vi "Rd Wr HK Settings.vi"(8 "error in (no error)":errorcluster, 9 "File Path":path, 10 "Write? (F:Read)":bool, 11 "channels":T1[](array[typedef])) -> (0 "error out":errorcluster, 3 "channels":T1[](array[typedef]))   [LabVIEW 2024, in "HK Table.lvclass"]
uses:
  HK Table.lvclass
  HK Channel Settings.ctl
  HK Item/HK Channel Units and Setup.ctl
  HK Item/HK Channel enum Data Type.ctl
  HK Item/HK Channel Settings Scaling.ctl
  HK Item/HK Channel enum Scaling Type.ctl
  HK Item/HK Channel Settings Physical.ctl
  HK Item/HK Channel Settings Limits.ctl
  HK Alarms/HK Channel Settings Alarms.ctl
  HK Alarms/HK Alarm enum Action.ctl
  5f5682ec-8197-494c-a0e5-daa0ddab1ed8.vi
  8967ee68-6fb9-484b-9a6b-7567600e0f71.vi
  <vilib>/JDP Science/JSONtext/JSON text to Variant.vi
  <vilib>/JDP Science/JSONtext/Variant to JSON Text.vi
  <vilib>/JDP Science/JSONtext/LVClass Serializer/JSONtext LVClass Serializer.lvclass
  HK Item/HK Item.lvclass
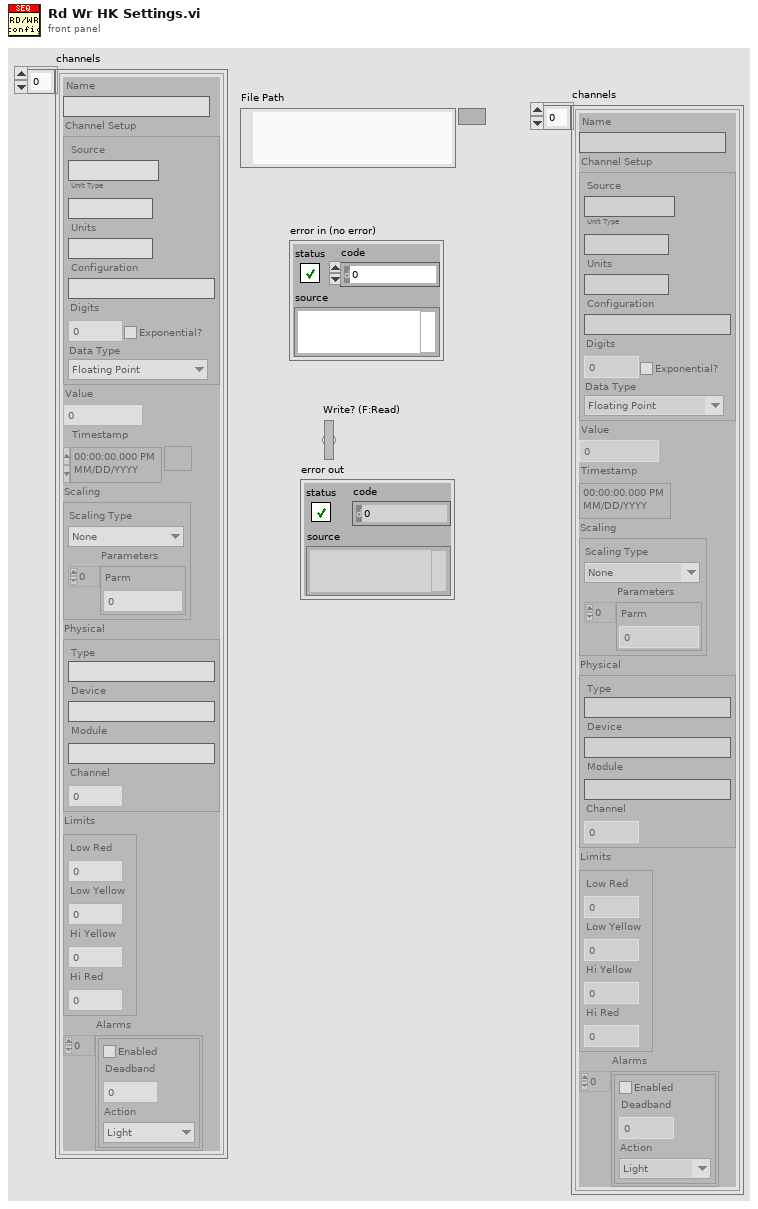
[diagram p1: front panel]
types:
  T1 = typedef "HK Table.lvclass/HK Channel Settings.ctl" = cluster{"Name":string, "Channel Setup":T2, "Value":dbl, "Timestamp":timestamp, "Scaling":T4, "Physical":T6, "Limits":T7, "Alarms":T8[]}
  T2 = typedef "HK Item.lvclass/HK Channel Units and Setup.ctl" = cluster{"Unit Type":string, "Units":string, "Configuration":string, "Digits":i32, "Data Type":T3, "Exponential?":bool, "Source":string}
  T3 = typedef "HK Item.lvclass/HK Channel enum Data Type.ctl" = enum16{"Floating Point", "Integer", "Enum", "String", "Waveform", "File"}
  T4 = typedef "HK Item.lvclass/HK Channel Settings Scaling.ctl" = cluster{"Scaling Type":T5, "Parameters":dbl[]}
  T5 = typedef "HK Item.lvclass/HK Channel enum Scaling Type.ctl" = enum16{"None", "Polynomial"}
  T6 = typedef "HK Item.lvclass/HK Channel Settings Physical.ctl" = cluster{"Type":string, "Device":string, "Module":string, "Channel":i32}
  T7 = typedef "HK Item.lvclass/HK Channel Settings Limits.ctl" = cluster{"Low Red":dbl, "Low Yellow":dbl, "Hi Yellow":dbl, "Hi Red":dbl}
  T8 = typedef "HK Item.lvclass/HK Channel Settings Alarms.ctl" = cluster{"Enabled":bool, "Deadband":i32, "Action":T9}
  T9 = typedef "HK Item.lvclass/HK Alarm enum Action.ctl" = enum16{"Light", "Message", "Safe"}
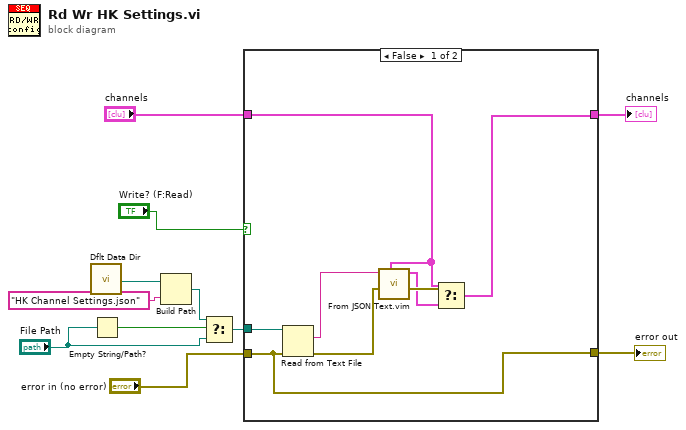
[diagram p0: block diagram]
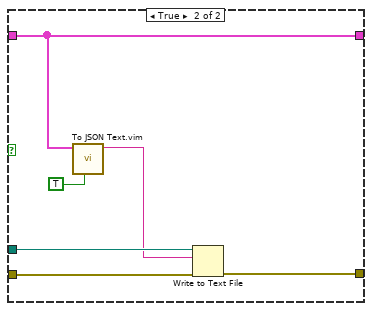
[diagram p2: hidden frame]
diagram:
  n1 = call <vilib>:"Dflt Data Dir.vi"() -> ("App:Default Data Directory"=w8:path)
  n2 = Empty String/Path?(string/path="File Path") -> (empty?=w4:bool)
  n3 = Build Path(base path=w8, name or relative path="HK Channel Settings.json") -> (appended path=w3:path)
  n4 = Select(t=w3, s=w4, f="File Path") -> (s? t:f=w1:path)
  n5 = case shown="False" "Write? (F:Read)" {
    tunnel: "error in (no error)" -> [w14 w25]
    tunnel: "channels" -> [w12 w22]
    tunnel: w1 -> [w19 w24]
    tunnel: [w14 w23] -> w7
    tunnel: [w15 w22] -> w6
    frame False {
      n6 = Read from Text File(file (use dialog)=w19, error in=w14) -> (text=w13:string, error out=w18:errorcluster)  [unwired: 2 in, 2 out]
      n7 = call "From JSON Text.vim"("Data Type and Default Value"=w12, "error in (no error)"=w18, "JSON"=w13) -> ("error out"=w17:errorcluster, "Data out"=w16:T1[])  [unwired: 7 in]
      n8 = Select(t=w12, s=w17, f=w16) -> (s? t:f=w15:T1[])
    }
    frame True {
      n9 = call "To JSON Text.vim"("Pretty Print?"=TRUE, "Anything"=w22) -> ("<JSON>"=w21:string)  [unwired: 8 in, 1 out]
      n10 = Write to Text File(file (use dialog)=w24, text=w21, error in=w25) -> (error out=w23:errorcluster)  [unwired: 1 in, 2 out]
    }
  }
  "error out" <- w7
  "channels" <- w6
